vi "Update_PM.vi"(7 "PM Modulation Cluster":T2={"Source (0: Internal)"=0, "Peak Deviation (90)"=90.0, "ON/OFF"=FALSE, "Modulation Frequency (10000)"=32467.5, "Modulation Waveform (1: Sine)"=1} {"Modulation Waveform (1: Sine)" items=["Sine"=1, "Square"=2, "Triangle"=3, "Ramp Up"=4, "Ramp Down"=5, "Noise"=100, "Arbitrary User1"=200, "Arbitrary User2"=201, "Arbitrary User3"=202, "Arbitrary User4"=203, "Edit Memory"=204]; "Source (0: Internal)" items=["Internal", "External"]}, 8 "error in (no error)":errorcluster {"code" format="%.0x"}, 10 "channel name (\"1\")":string="1", 11 "resource name":refnum<k15>) -> (0 "error out":errorcluster {"code" format="%.0x"}, 2 "output cluster":T1, 3 "instrument handle out":refnum<k15>)   [LabVIEW 2015, in "MyToolsFunction.lvlib"]
uses:
  ICcamera/MyToolsFunction.lvlib
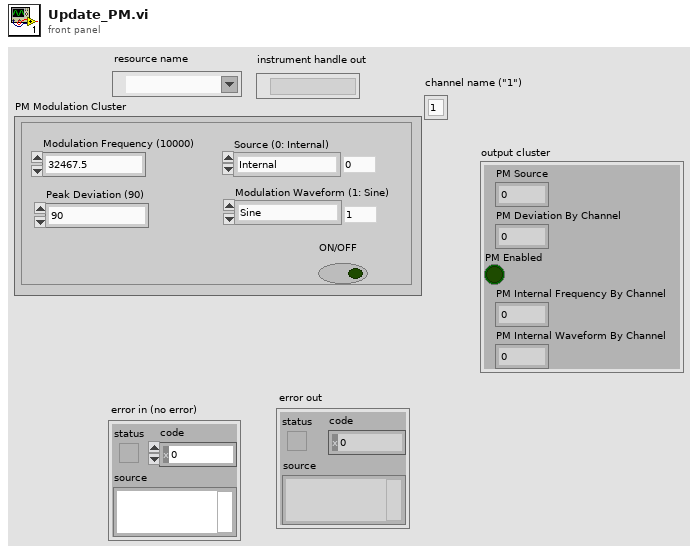
[diagram p1: front panel]
types:
  T1 = cluster{"PM Source":i32, "PM Deviation By Channel":dbl, "PM Enabled":bool, "PM Internal Frequency By Channel":dbl, "PM Internal Waveform By Channel":i32}
  T2 = cluster{"Source (0: Internal)":i32, "Peak Deviation (90)":dbl, "ON/OFF":bool, "Modulation Frequency (10000)":dbl, "Modulation Waveform (1: Sine)":i32}
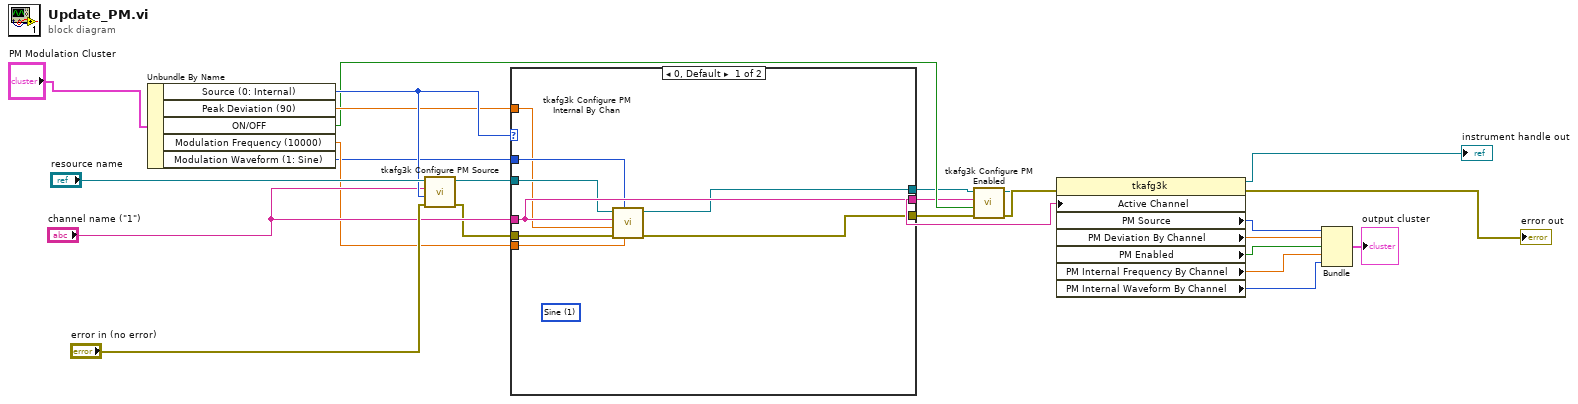
[diagram p0: block diagram]
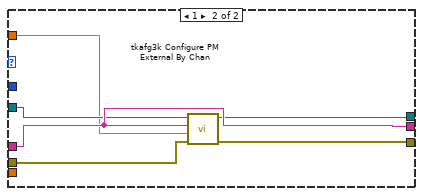
[diagram p2: hidden frame]
diagram:
  n1 = Unbundle By Name("PM Modulation Cluster") -> ("Source (0: Internal)"=w22:i32, "Peak Deviation (90)"=w21:dbl, "ON/OFF"=w20:bool, "Modulation Frequency (10000)"=w14:dbl, "Modulation Waveform (1: Sine)"=w12:i32)
  n2 = call <instrlib>:"tkafg3k Configure PM Source.vi"("error in (no error)"="error in (no error)", "Source (0: Internal)"=w22, "Channel Name (\"1\")"="channel name (\"1\")", "instrument handle"="resource name") -> ("error out"=w18:errorcluster, "instrument handle out"=w16:refnum<k15>)  [unwired: 6 in]
  n3 = case shown="0, Default" w22 {
    tunnel: w21 -> [w25 w33]
    tunnel: "channel name (\"1\")" -> [w30 w36]
    tunnel: w18 -> [w32 w38]
    tunnel: [w31 w37] -> w17
    tunnel: [w30 w36] -> w11
    tunnel: w16 -> [w29 w35]
    tunnel: [w28 w34] -> w15
    tunnel: w14 -> [w27 _]
    tunnel: w12 -> [w26 _]
    frame 0, Default {
      (unwired) 1 items=["Sine"=1, "Square"=2, "Triangle"=3, "Ramp Up"=4, "Ramp Down"=5, "Noise"=100, "Arbitrary User1"=200, "Arbitrary User2"=201, "Arbitrary User3"=202, "Arbitrary User4"=203, "Edit Memory"=204] ("Modulation Waveform (1: Sine)")
      n4 = call <instrlib>:"tkafg3k Configure PM Internal By Chan.vi"("Modulation Frequency (10000)"=w27, "Modulation Waveform (1: Sine)"=w26, "error in (no error)"=w32, "Peak Deviation (90)"=w25, "Channel Name (\"1\")"=w30, "instrument handle"=w29) -> ("error out"=w31:errorcluster, "instrument handle out"=w28:refnum<k15>)  [unwired: 4 in]
    }
    frame 1 {
      n5 = call <instrlib>:"tkafg3k Configure PM External By Chan.vi"("error in (no error)"=w38, "Peak Deviation (90)"=w33, "Channel Name (\"1\")"=w36, "instrument handle"=w35) -> ("error out"=w37:errorcluster, "instrument handle out"=w34:refnum<k15>)  [unwired: 6 in]
    }
  }
  n6 = call <instrlib>:"tkafg3k Configure PM Enabled.vi"("error in (no error)"=w17, "Enabled (True)"=w20, "Channel Name (\"1\")"=w11, "instrument handle"=w15) -> ("error out"=w10:errorcluster, "instrument handle out"=w8:refnum<k15>)  [unwired: 6 in]
  n7 = property class="tkafg3k"(reference=w8, error in=w10, "Active Channel"=w11) -> (reference out=→"instrument handle out":refnum<k15>, error out=→"error out":errorcluster, "PM Source"=w6:i32, "PM Deviation By Channel"=w5:dbl, "PM Enabled"=w4:bool, "PM Internal Frequency By Channel"=w3:dbl, "PM Internal Waveform By Channel"=w2:i32)
  n8 = Bundle("PM Source"=w6, "PM Deviation By Channel"=w5, "PM Enabled"=w4, "PM Internal Frequency By Channel"=w3, "PM Internal Waveform By Channel"=w2) -> (→"output cluster":T1)  [unwired: 1 in]
